vi "Set Intensity Graph X Scale Array.vi"(8 "error in (no error)":errorcluster, 10 "X Scale":dbl[](array[numeric]), 11 "graph_utilities in":refnum<class "graph_utilities.lvclass">) -> (0 "error out":errorcluster, 3 "graph_utilities out":refnum<class "graph_utilities.lvclass">)   [LabVIEW 2020, in "graph_utilities.lvclass"]
doc: "Set the X Offset and Multiple of the Intensity Graph by wiring an array to X Scale"
uses:
  graph_utilities.lvclass
  graph_utilities.lvclass/graph_utilities.ctl
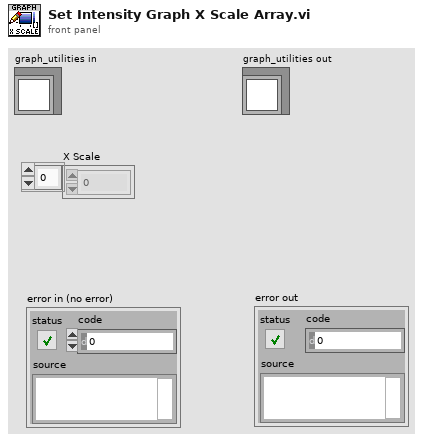
[diagram p1: front panel]
types:
  T1 = typedef "LVOffsetAndMultiplierTypeDef.ctl" = cluster{"Offset":dbl, "Multiplier":dbl}
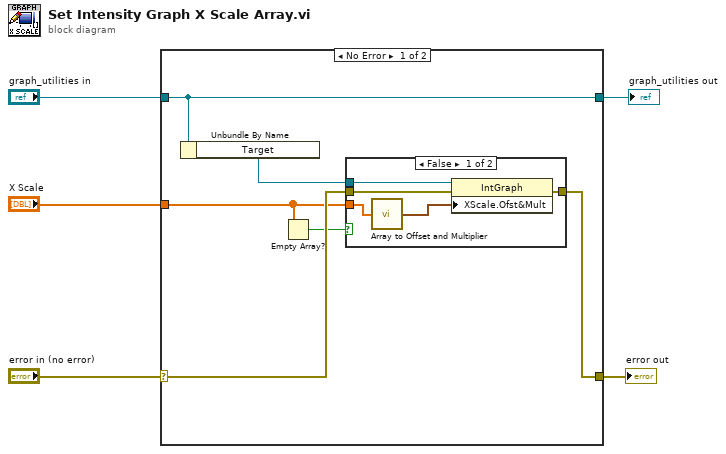
[diagram p0: block diagram]
diagram:
  n1 = case shown="No Error" "error in (no error)" {
    selector: "error in (no error)" -> [w10 w19]
    tunnel: "X Scale" -> [w6 _]
    tunnel: [w11 w19] -> w4
    tunnel: "graph_utilities in" -> [w9 w18]
    tunnel: [w9 w18] -> w1
    frame No Error {
      n2 = Unbundle By Name(w9) -> ("Target"=w8:refnum<vi>)
      n3 = Empty Array?(array=w6) -> (empty?=w7:bool)
      n4 = case shown="False" w7 {
        tunnel: [w16 w17] -> w11
        tunnel: w10 -> [w15 w17]
        tunnel: w8 -> [w14 _]
        tunnel: w6 -> [w12 _]
        frame False {
          n5 = call "Array to Offset and Multiplier.vi"("Array"=w12) -> ("Offset and Multiplier"=w13:T1)
          n6 = property on="Property Node" class="IntGraph"(reference=w14, error in=w15, "XScale.Ofst&Mult"=w13) -> (error out=w16:errorcluster)  [unwired: 1 out]
        }
        frame True {
        }
      }
    }
    frame Error {
    }
  }
  "error out" <- w4
  "graph_utilities out" <- w1
